vi "Draw Overlay Point.vi"(9 "Color":u32(colorbox)=16711680, 10 "Cluster":cluster{"Position.X":dbl, "Position.Y":dbl}, 11 "Refnum in":T1) -> (3 "Refnum out":T1)   [LabVIEW 2019]
uses:
  <vilib>/vision/Image Controls.llb/IMAQ Image.ctl
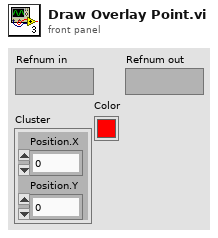
[diagram p1: front panel]
types:
  T1 = typedef "IMAQ Image.ctl" = refnum<image>
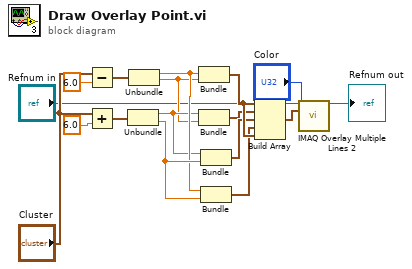
[diagram p0: block diagram]
diagram:
  n1 = Subtract(x="Cluster", y=6.0) -> (x-y=w5:cluster{"Position.X":dbl, "Position.Y":dbl})
  n2 = Add(x="Cluster", y=6.0) -> (x+y=w6:cluster{"Position.X":dbl, "Position.Y":dbl})
  n3 = Unbundle(w6) -> ("Position.X"=w8:dbl, "Position.Y"=w10:dbl)
  n4 = Unbundle(w5) -> ("Position.X"=w9:dbl, "Position.Y"=w7:dbl)
  n5 = Bundle("Position.X"=w9, "Position.Y"=w7) -> (w14:cluster{"Position.X":dbl, "Position.Y":dbl})  [unwired: 1 in]
  n6 = Bundle("Position.X"=w8, "Position.Y"=w7) -> (w11:cluster{"Position.X":dbl, "Position.Y":dbl})  [unwired: 1 in]
  n7 = Bundle("Position.X"=w8, "Position.Y"=w10) -> (w12:cluster{"Position.X":dbl, "Position.Y":dbl})  [unwired: 1 in]
  n8 = Bundle("Position.X"=w9, "Position.Y"=w10) -> (w13:cluster{"Position.X":dbl, "Position.Y":dbl})  [unwired: 1 in]
  n9 = Build Array(w14, w11, w12, w13, w14) -> (w15:cluster{"Position.X":dbl, "Position.Y":dbl}[])
  n10 = call "IMAQ Overlay Multiple Lines 2"("Image"="Refnum in", "Line End Points"=w15, "Color"="Color") -> ("Image Out"=→"Refnum out":T1)  [unwired: 11 in, 1 out]
